vi "setUp.vi"(8 "error in (no error)":errorcluster, 11 "reference in":refnum<class "Test Nested Endpoint Transmit Failure.lvclass">) -> (0 "error out":errorcluster, 3 "reference out":refnum<class "Test Nested Endpoint Transmit Failure.lvclass">)   [LabVIEW 2020, in "Test Nested Endpoint Transmit Failure.lvclass"]
doc: "setUp runs prior to the test method during test execution. Use this method to initialize any object data required by your tests."
uses:
  Test Nested Endpoint Transmit Failure.lvclass
  <vilib>/addons/_JKI Toolkits/VI Tester/TestCase.llb/TestCase.lvclass
  <vilib>/ActorFramework/Actor/Actor.lvclass
  <vilib>/ActorFramework/Message Queue/Message Queue.lvclass
  Source/Nested Endpoint/Nested Endpoint/Nested Endpoint.lvclass
  Source/Network Endpoint/Network Endpoint/Network Endpoint.lvclass
  Support/Error Stream/Error Stream.lvclass
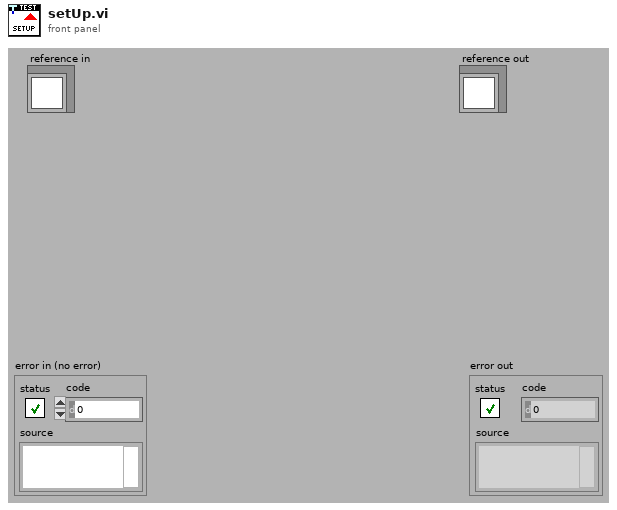
[diagram p1: front panel]
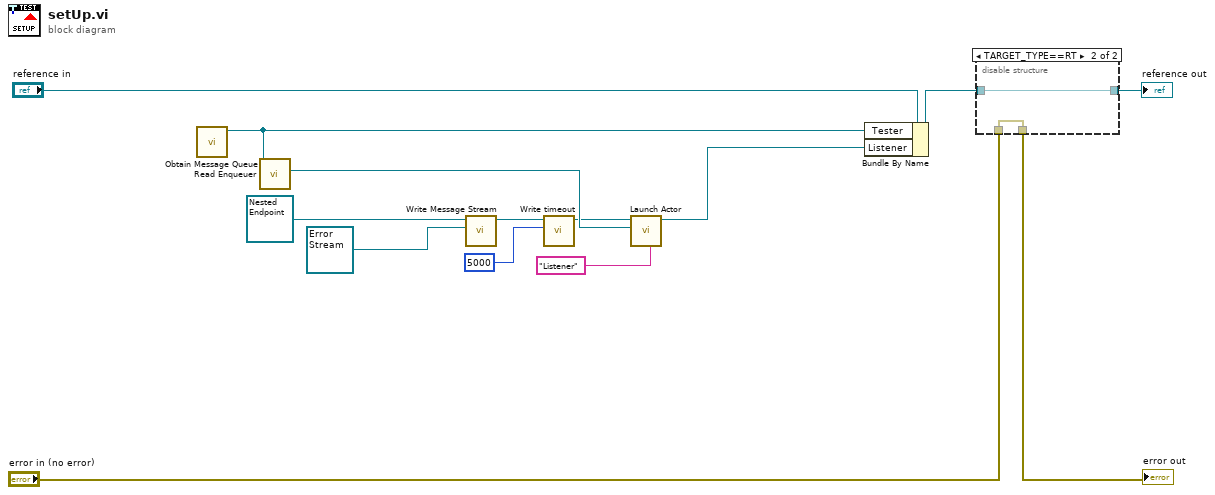
[diagram p0: block diagram]
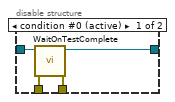
[diagram p2: hidden frame]
diagram:
  n1 = call <vilib>:"Obtain Message Queue.vi"() -> ("Message Queue"=w6:refnum<class "Message Queue.lvclass">)  [unwired: 10 in, 1 out]
  n2 = call <vilib>:"Read Enqueuer.vi"("Message Queue"=w6) -> ("Message Enqueuer"=w10:refnum<class "Message Enqueuer.lvclass">)  [unwired: 10 in]
  n3 = call "Write Message Stream.vi"("Message Stream"=refnum<class "Error Stream.lvclass"> refnum ("Error Stream.lvclass"), "Network Endpoint in"=refnum<class "Nested Endpoint.lvclass"> refnum ("Nested Endpoint.lvlib:Nested Endpoint.lvclass")) -> ("Network Endpoint out"=w5:refnum<class "Nested Endpoint.lvclass">)  [unwired: 9 in]
  n4 = call "Write timeout.vi"("timeout"=5000, "Network Endpoint in"=w5) -> ("Network Endpoint out"=w4:refnum<class "Nested Endpoint.lvclass">)  [unwired: 9 in]
  n5 = call <vilib>:"Launch Actor.vi"("Debug Alias"="Listener", "Actor-to-Caller Enqueuer"=w10, "Actor"=w4) -> ("Caller-To-Actor Enqueuer"=w7:refnum<class "Message Enqueuer.lvclass">)  [unwired: 7 in, 1 out]
  n6 = Bundle By Name(cluster="reference in", "Tester"=w6, "Listener"=w7) -> (w11:refnum<class "Test Nested Endpoint Transmit Failure.lvclass">)
  n7 = disable-structure shown="TARGET_TYPE==RT" {
    disable-tunnel: "error in (no error)" -> [w18 w19]
    disable-tunnel: [w17 w19] -> w14
    disable-tunnel: [w16 w20] -> w12
    disable-tunnel: w11 -> [w15 w20]
    frame condition #0 (active) {
      n8 = call <vilib>:"WaitOnTestComplete.vi"("error in (no error)"=w18, "TestCase in"=w15) -> ("error out"=w17:errorcluster, "TestCase out"=w16:refnum<class "Test Nested Endpoint Transmit Failure.lvclass">)  [unwired: 8 in]
    }
    frame condition #1 {
    }
  }
  "error out" <- w14
  "reference out" <- w12
